vi "MaxHeapify.vi"(8 "Error in (no error)":errorcluster, 9 "Length":i32, 10 "i":i32, 11 "Heap in":refnum<class "UintClass.lvclass">[](array[class])) -> (0 "Error out":errorcluster, 3 "Heap out":refnum<class "UintClass.lvclass">[](array[class]))   [LabVIEW 2011, in "UintClass.lvclass"]
uses:
  UintClass.lvclass
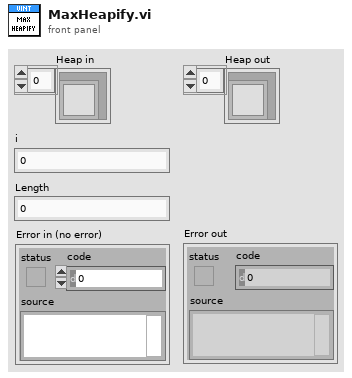
[diagram p1: front panel]
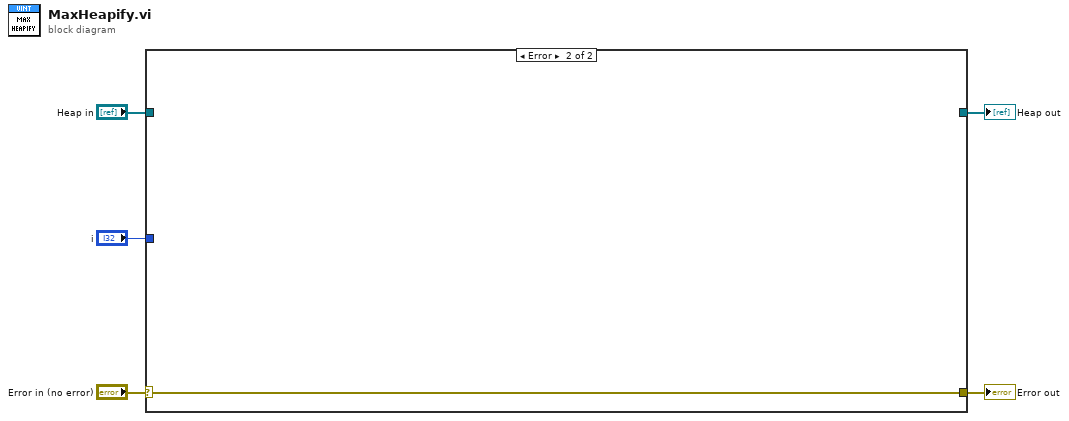
[diagram p0: block diagram]
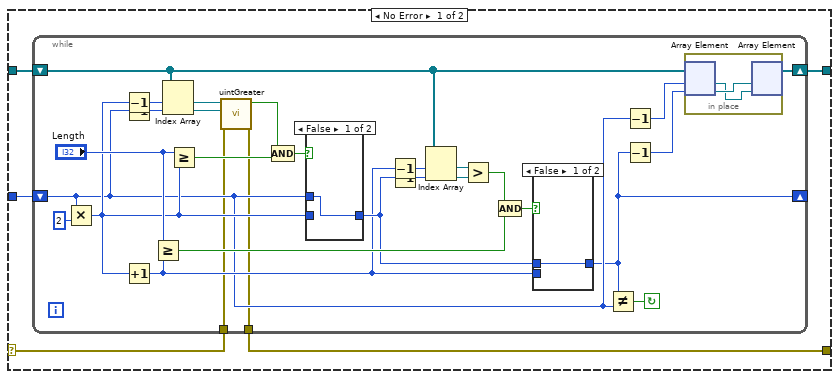
[diagram p2: hidden frame]
diagram:
  n1 = case shown="Error" "Error in (no error)" {
    selector: "Error in (no error)" -> [w6 w45]
    tunnel: "Heap in" -> [w10 _]
    tunnel: [w9 _] -> w4
    tunnel: "i" -> [w8 _]
    tunnel: [w7 w45] -> w2
    frame No Error {
      n2 = while {
        shift-right: [w14] -> w9
        shift-left: w10 -> [w15]
        shift-right: [w20] -> _
        shift-left: w8 -> [w21]
        tunnel: w6 -> [w17]
        tunnel: [w16] -> w7
        stop <- w25 continue-if-true
        n3 = Multiply(x=w21, y=2 ("x")) -> (x*y=w24:i32)
        n4 = Decrement(x=w24) -> (x-1=w31:i32)
        n5 = Decrement(x=w21) -> (x-1=w30:i32)
        n6 = Increment(x=w24) -> (x+1=w23:i32)
        n7 = Greater Or Equal?(x="Length", y=w23) -> (x >= y?=w33:bool)
        n8 = Index Array(array=w15, index #1=w31, index #2=w30) -> (element #1=w19:refnum<class "UintClass.lvclass">, element #2=w18:refnum<class "UintClass.lvclass">)
        n9 = Greater Or Equal?(x="Length", y=w24) -> (x >= y?=w38:bool)
        n10 = call "uintGreater.vi"("Error in (no error)"=w17, "Int2 in"=w18, "Int1 in"=w19) -> ("Error out"=w16:errorcluster, "Int1 > Int2?"=w11:bool)  [unwired: 6 in, 1 out]
        n11 = Compound Arithmetic op=AND(w11, w38) -> (w37:bool)
        n12 = case shown="False" w37 {
          tunnel: w24 -> [_ w44]
          tunnel: w21 -> [w43 _]
          tunnel: [w43 w44] -> w27
          frame False {
          }
          frame True {
          }
        }
        n13 = Decrement(x=w23) -> (x-1=w28:i32)
        n14 = Decrement(x=w27) -> (x-1=w29:i32)
        n15 = Index Array(array=w15, index #1=w28, index #2=w29) -> (element #1=w35:refnum<class "UintClass.lvclass">, element #2=w36:refnum<class "UintClass.lvclass">)
        n16 = Greater?(x=w35, y=w36) -> (0:w32:bool)
        n17 = Compound Arithmetic op=AND(w32, w33) -> (w34:bool)
        n18 = case shown="False" w34 {
          tunnel: w27 -> [w41 _]
          tunnel: w23 -> [_ w42]
          tunnel: [w41 w42] -> w20
          frame False {
          }
          frame True {
          }
        }
        n19 = Not Equal?(x=w20, y=w21) -> (x != y?=w25:bool)
        n20 = Decrement(x=w21) -> (x-1=w13:i32)
        n21 = Decrement(x=w20) -> (x-1=w12:i32)
        n22 = in-place {
          n23 = in-place-array #1(w15, w13, w12) -> (w39:refnum<class "UintClass.lvclass">, w40:refnum<class "UintClass.lvclass">)
          n24 = in-place-array #1(w40, w39) -> (w14:refnum<class "UintClass.lvclass">[])  [unwired: 2 out]
        }
      }
    }
    frame Error {
    }
  }
  "Heap out" <- w4
  "Error out" <- w2
